vi "Calculate Correct Speed.vi"(10 "Desired Speed":dbl, 11 "Pivot":enum16{"FL", "FR", "BL", "BR"}(ring)) -> (3 "Correct Speed":dbl)   [LabVIEW 2014]
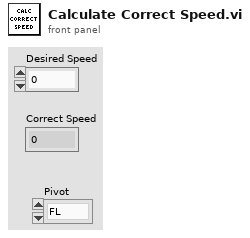
[diagram p1: front panel]
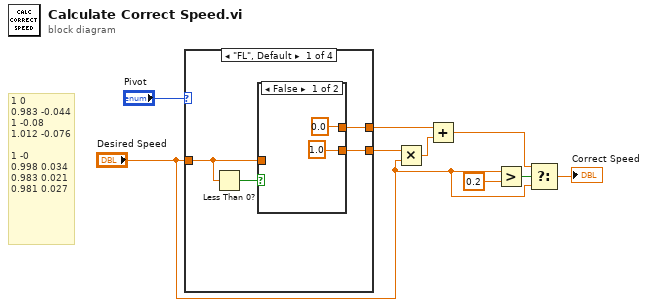
[diagram p0: block diagram]
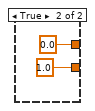
[diagram p2: hidden frame]
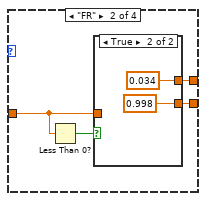
[diagram p3: hidden frame]
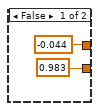
[diagram p4: hidden frame]
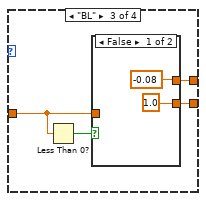
[diagram p5: hidden frame]
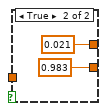
[diagram p6: hidden frame]
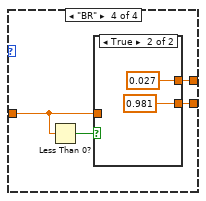
[diagram p7: hidden frame]
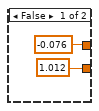
[diagram p8: hidden frame]
diagram:
  # "1\t0\n0.983\t-0.044\n1\t-0.08\n1.012\t-0.076\n\n1\t-0\n0.998\t0.034\n0.983\t0.021\n0.981\t0.027"
  n1 = case shown="\"FL\", Default" "Pivot" {
    tunnel: "Desired Speed" -> [w12 w20 w28 w36]
    tunnel: [w11 w19 w27 w34] -> w7
    tunnel: [w10 w18 w26 w35] -> w6
    frame "FL", Default {
      n2 = Less Than 0?(x=w12) -> (x < 0?=w13:bool)
      n3 = case shown="False" w13 {
        tunnel: w12 -> [_ _]
        tunnel: [0.0 ("x") 0.0 ("x")] -> w11
        tunnel: [1.0 ("x") 1.0 ("x")] -> w10
        frame False {
        }
        frame True {
        }
      }
    }
    frame "FR" {
      n4 = Less Than 0?(x=w20) -> (x < 0?=w21:bool)
      n5 = case shown="True" w21 {
        tunnel: w20 -> [_ _]
        tunnel: [-0.044 ("x") 0.034 ("x")] -> w19
        tunnel: [0.983 ("x") 0.998 ("x")] -> w18
        frame False {
        }
        frame True {
        }
      }
    }
    frame "BL" {
      n6 = Less Than 0?(x=w28) -> (x < 0?=w29:bool)
      n7 = case shown="False" w29 {
        tunnel: w28 -> [_ _]
        tunnel: [-0.08 ("x") 0.021 ("x")] -> w27
        tunnel: [1.0 ("x") 0.983 ("x")] -> w26
        frame False {
        }
        frame True {
        }
      }
    }
    frame "BR" {
      n8 = Less Than 0?(x=w36) -> (x < 0?=w37:bool)
      n9 = case shown="True" w37 {
        tunnel: w36 -> [_ _]
        tunnel: [-0.076 ("x") 0.027 ("x")] -> w34
        tunnel: [1.012 ("x") 0.981 ("x")] -> w35
        frame False {
        }
        frame True {
        }
      }
    }
  }
  n10 = Multiply(x=w6, y="Desired Speed") -> (x*y=w8:dbl)
  n11 = Add(x=w7, y=w8) -> (x+y=w2:dbl)
  n12 = Greater?(x="Desired Speed", y=0.2) -> (0:w4:bool)
  n13 = Select(t=w2, s=w4, f="Desired Speed") -> (s? t:f=→"Correct Speed":dbl)
